vi "runTestScenario.vi"(8 "error in (no error)":errorcluster, 11 "3.3VDSupplyTest in":refnum<class "+3.3VDSupplyTest.lvclass">) -> (0 "error out":errorcluster, 2 "TestExecution":T1, 3 "3.3VDSupplyTest out":refnum<class "+3.3VDSupplyTest.lvclass">)   [LabVIEW 2015, in "+3.3VDSupplyTest.lvclass"]
uses:
  +3.3VDSupplyTest.lvclass
  Typedefs/TestExecution.ctl
  Typedefs/WriteDataFileInput.ctl
  Typedefs/TestScenarioTypes.ctl
  Typedefs/WriteLogMessageInput.ctl
  Typedefs/PassFailTest.ctl
  +3.3VDSupplyTest.lvclass/+3.3VDSupplyTest.ctl
  Model/TestLog/ITestLog/ITestLog.lvclass
  Typedefs/ILCBTTypedefs.lvlib
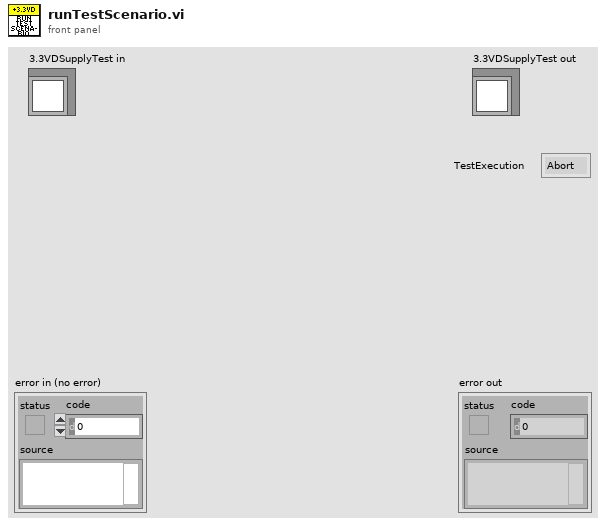
[diagram p1: front panel]
types:
  T1 = typedef "ILCBTTypedefs.lvlib/TestExecution.ctl" = enum16{"Abort", "Continue"}
  T2 = typedef "ILCBTTypedefs.lvlib/WriteLogMessageInput.ctl" = cluster{"Test Scenario":T3, "Description":string, "Actual Value":string, "Data File":string, "Result":T4}
  T3 = typedef "ILCBTTypedefs.lvlib/TestScenarioTypes.ctl" = enum16{"+3.3VA Supply Test", "+3.3VD Supply Test", "+5VA Supply Test", "+5VD Supply Test"}
  T4 = typedef "ILCBTTypedefs.lvlib/PassFailTest.ctl" = enum16{"Fail", "Pass", "NA"}
  T5 = typedef "ILCBTTypedefs.lvlib/WriteDataFileInput.ctl" = cluster{"Test Scenario":T3, "File Name":string, "Output":dbl[]}
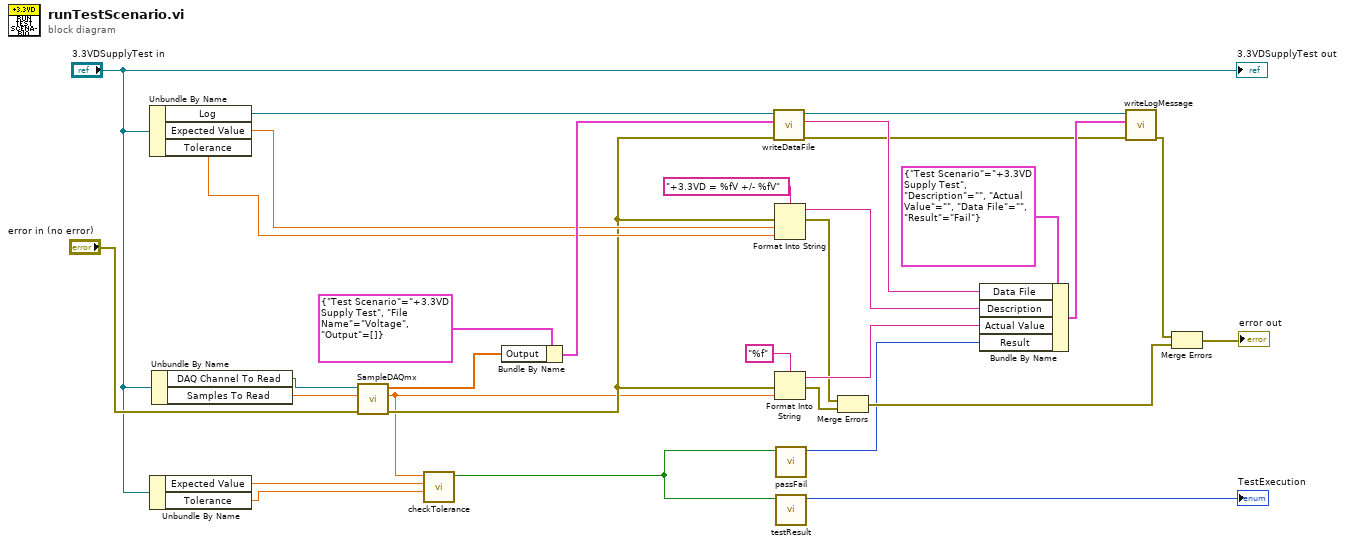
[diagram p0: block diagram]
diagram:
  n1 = Unbundle By Name("3.3VDSupplyTest in") -> ("Log"=w30:refnum<class "ITestLog.lvclass">, "Expected Value"=w19:dbl[unit], "Tolerance"=w18:dbl[unit])
  n2 = Unbundle By Name("3.3VDSupplyTest in") -> ("Expected Value"=w5:dbl[unit], "Tolerance"=w1:dbl[unit])
  n3 = Unbundle By Name("3.3VDSupplyTest in") -> ("DAQ Channel To Read"=w23:refnum<k21>, "Samples To Read"=w22:dbl)
  n4 = call "SampleDAQmx.vi"("error in (no error)"="error in (no error)", "Samples To Read"=w22, "DAQ Channel To Read"=w23) -> ("error out"=w17:errorcluster, "Average"=w6:dbl, "Samples"=w29:dbl[])  [unwired: 6 in]
  n5 = call "checkTolerance.vi"("Tolerance"=w1, "Expected Value"=w5, "Average"=w6) -> ("Boolean"=w4:bool)  [unwired: 8 in]
  n6 = Bundle By Name(cluster=T5 {"Test Scenario"=enum."+3.3VD Supply Test", "File Name"="Voltage", "Output"=[]} ("WriteDataFileInput"), "Output"=w29) -> (w20:T5)
  n7 = call-dynamic "writeDataFile.vi"("error in (no error)"=w17, "WriteDataFileInput"=w20, "ITestLog in"=w30) -> ("error out"=w13:errorcluster, "Relative Path"=w16:string, "ITestLog out"=w25:refnum<class "ITestLog.lvclass">)  [unwired: 6 in]
  n8 = Format Into String(format string="+3.3VD = %fV +/- %fV", error in=w17, w19, w18) -> (resulting string=w15:string, error out=w12:errorcluster)  [unwired: 1 in]
  n9 = Format Into String(format string="%f", error in=w17, w6) -> (resulting string=w14:string, error out=w11:errorcluster)  [unwired: 1 in]
  n10 = call "passFail.vi"("Boolean"=w4) -> ("Result"=w2:T4)  [unwired: 10 in]
  n11 = call "testResult.vi"("Boolean"=w4) -> ("TestExecution"=→"TestExecution":T1)  [unwired: 10 in]
  n12 = Merge Errors(w12, w11) -> (w8:errorcluster)
  n13 = Bundle By Name(cluster=T2 {"Test Scenario"=enum."+3.3VD Supply Test", "Description"="", "Actual Value"="", "Data File"="", "Result"=enum."Fail"} ("WriteLogMessageInput"), "Data File"=w16, "Description"=w15, "Actual Value"=w14, "Result"=w2) -> (w24:T2)
  n14 = call-dynamic "writeLogMessage.vi"("error in (no error)"=w13, "WriteLogMessageInput"=w24, "ITestLog in"=w25) -> ("error out"=w9:errorcluster)  [unwired: 7 in, 1 out]
  n15 = Merge Errors(w9, w8) -> (→"error out":errorcluster)
  "3.3VDSupplyTest out" <- "3.3VDSupplyTest in"
